vi "Mass_1_3.vi"() -> ()   [LabVIEW 2020]
uses:
  Support/Controls/Cmd_Mouse Popup.ctl
  Support/Controls/Clst_Initialize Input.ctl
  Support/Controls/Clst_Result inspec.ctl
  Support/Controls/Cmd_Var Data IO.ctl
  Variables/Global_Cal Info.vi
panel:
  in  "Measured_ADJ":string[][](table) caption="저울의 지시값 (조정후)"
  out "분동조합":string[][](table)
  in  "Spec 변경":bool
  in  "Random":bool
  out "Spec":string[][](table)
  out "제목":string
  out "편심 오차 시험 분동":string
  out "에러 출력":errorcluster
  out "Condition":string[][](table) caption="2. 직선성 시험"
  in  "최소눈금":string(combo)
  out "단위":string
  out "최대용량":string
  in  "Measured":string[][](table) caption="저울의 지시값"
  in  "Measured 2":string[][](table) caption="1. 편심오차 시험"
  out "Load?":bool
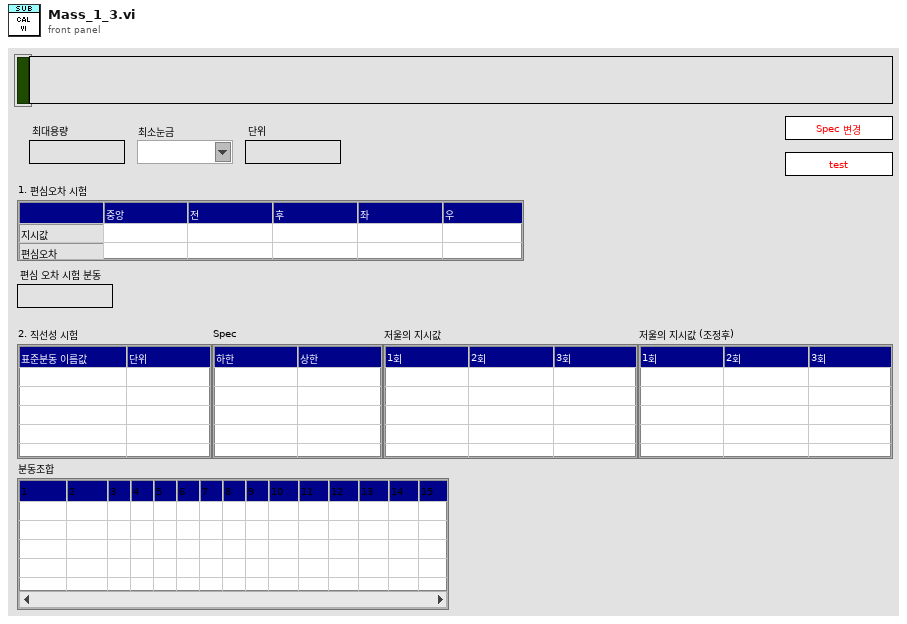
[diagram p1: front panel]
types:
  T1 = typedef "Cmd_Mouse Popup.ctl" = enum16{"활성화", "메뉴선택"}
  T2 = cluster{"Shift":bool, "Ctrl":bool, "Alt":bool, "Cmd":bool, "Opt":bool}
  T3 = typedef "Clst_Initialize Input.ctl" = cluster{"Initialize 1":cluster{"Condition":refnum<vi>[], "Spec":refnum<vi>[], "Measured":refnum<vi>[], "Resolution":refnum<vi>[], "Func_ext":string, "제목":refnum<vi>, "Measured_ADJ":refnum<vi>[]}, "Initialize 2":cluster{"문자열":refnum<vi>[], "콤보박스":refnum<vi>[], "링":refnum<vi>[], "열거형":refnum<vi>[], "테이블":refnum<vi>[], "여러열":refnum<vi>[], "디지털(DBL)":refnum<vi>[], "3D string":refnum<vi>[], "ctrl":refnum<vi>[], "boolean":refnum<vi>[]}}
  T4 = typedef "Clst_Result inspec.ctl" = cluster{"분해능":string, "문자열 1":string, "문자열 2":string, "숫자형 1":i32, "숫자형 2":i32, "숫자형 3":dbl, "문자배열 1D":string[], "문자배열 2D":string[][], "문자배열 3D":string[][][], "문자배열 4D":string[][][][], "불리언 1D":bool[]}
  T5 = typedef "Cmd_Var Data IO.ctl" = enum16{"Condition", "Condition Default", "Condition_Temp", "Resolution", "Resolution Default", "Resolution Old", "Spec", "Spec Default", "Spec Old", "Spec Temp", "Result", "Result2", "Result3", "Result_Temp", "Result_ADJ", "Result_ADJ2", "STD1", "STD2", "STD3", "STD4", "STD5", "STD Temp", "CMC", "CMC Default"}
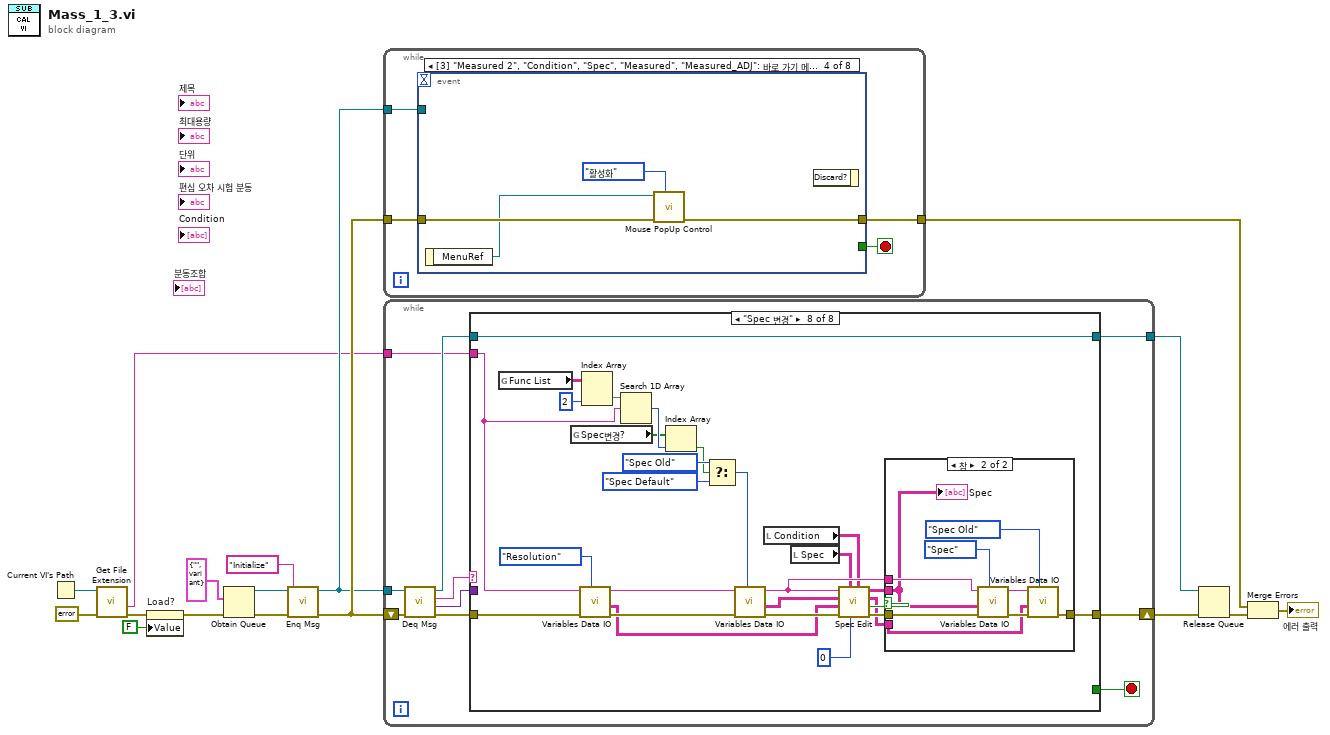
[diagram p0: block diagram]
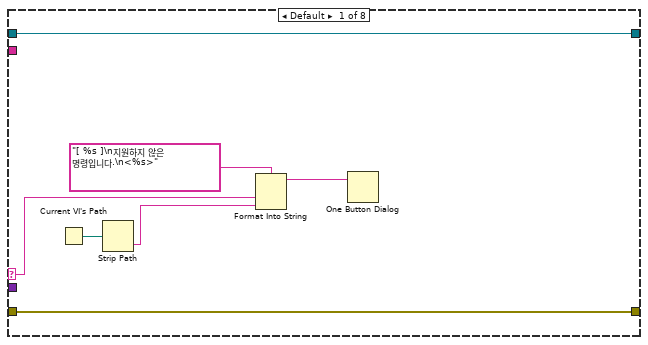
[diagram p2: hidden frame]
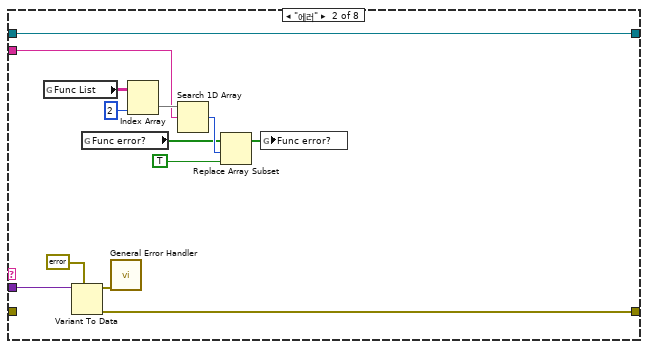
[diagram p3: hidden frame]
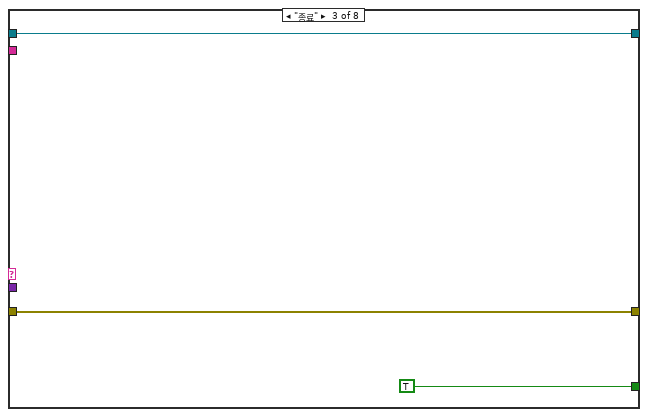
[diagram p4: hidden frame]
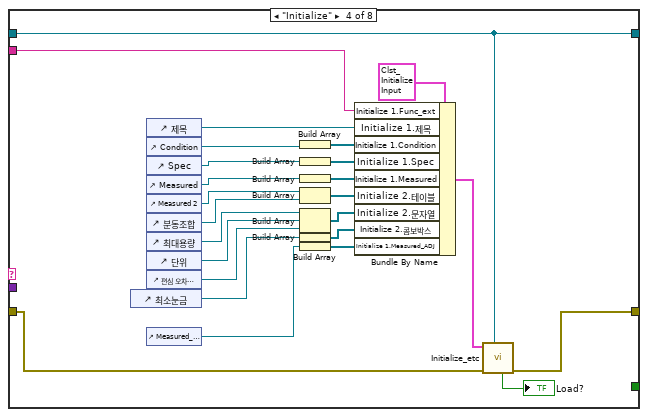
[diagram p5: hidden frame]
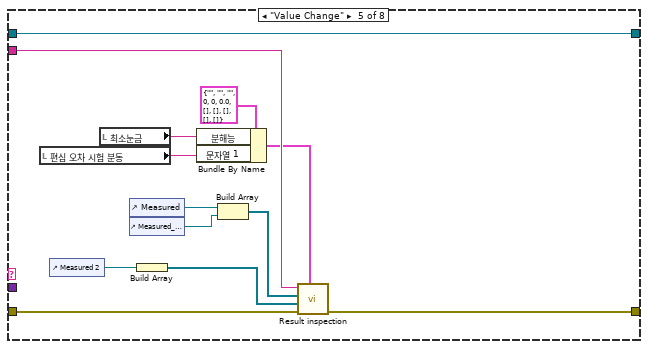
[diagram p6: hidden frame]
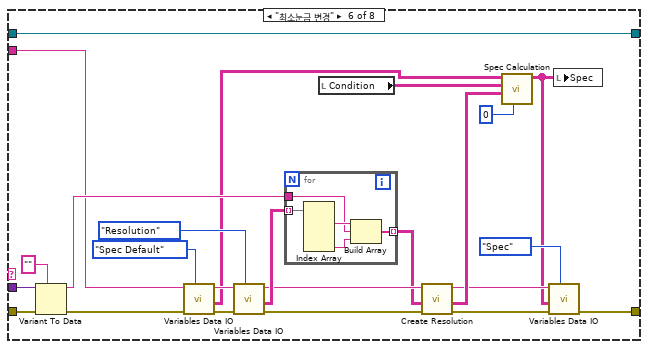
[diagram p7: hidden frame]
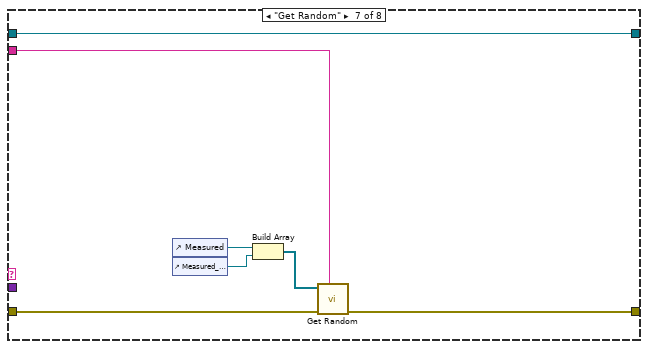
[diagram p8: hidden frame]
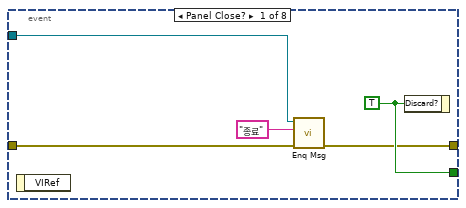
[diagram p10: hidden frame]
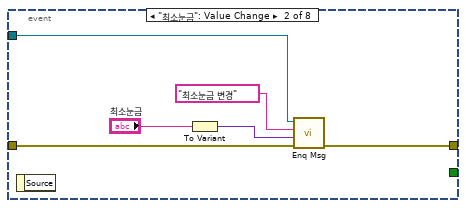
[diagram p11: hidden frame]
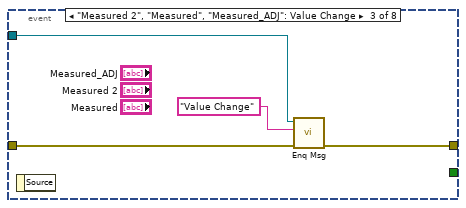
[diagram p12: hidden frame]
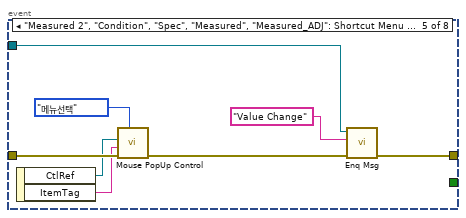
[diagram p13: hidden frame]
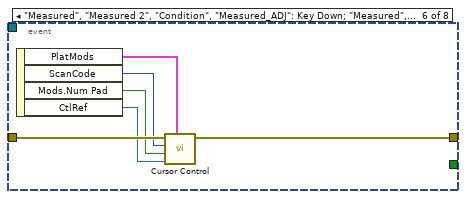
[diagram p14: hidden frame]
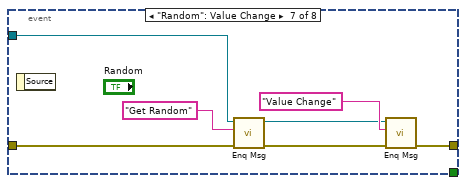
[diagram p15: hidden frame]
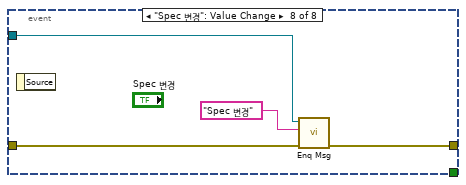
[diagram p16: hidden frame]
diagram:
  n1 = Current VI's Path() -> (path=w5:path)
  n2 = call <vilib>:"Get File Extension.vi"("error in (no error)"=errorcluster {"status"=FALSE, "code"=0, "source"=""} ("에러 상수"), "file"=w5) -> ("error out"=w3:errorcluster, "filename without extension"=w4:string)  [unwired: 5 in, 3 out]
  n3 = property on="Load?" class="Bool (엄격한)"(error in=w3, "Value"=FALSE ("Load?")) -> (error out=w2:errorcluster)  [unwired: 1 in, 1 out]
  n4 = Obtain Queue(element data type=cluster{"메세지":string, "값":variant} {"메세지"="", "값"=variant} ("Message Cluster"), error in (no error)=w2) -> (queue out=w14:refnum<queue>, error out=w16:errorcluster)  [unwired: 3 in, 1 out]
  n5 = call "Enq Msg.vi"("에러 입력(에러 없음)"=w16, "메세지"="Initialize", "큐 입력"=w14) -> ("에러 출력"=w15:errorcluster, "큐 출력"=w12:refnum<queue>)  [unwired: 7 in]
  n6 = while {
    tunnel: w15 -> [w19]
    tunnel: w12 -> [w20]
    tunnel: [w18] -> w9
    stop <- w21 stop-if-true
    n7 = event shown="[3] \"Measured 2\", \"Condition\", \"Spec\", \"Measured\", \"Measured_ADJ\": 바로 가기 메뉴 활성화?" {
      selector: _ -> [_ _ _ _ _ _ _ _]
      dyn-events: _ -> [_ _ _ _ _ _ _ _]
      timeout: _ -> [_ _ _ _ _ _ _ _]
      tunnel: [w26 _ _ _ _ _ _ _] -> w21
      tunnel: w20 -> [w24 w31 w35 _ w42 _ w56 w62]
      tunnel: w19 -> [w25 w32 w36 w39 w47 w54 w57 w64]
      tunnel: [w22 w29 w33 w38 w41 w53 w55 w63] -> w18
      event Panel Close? {
        w26 = TRUE ("버림?")
        n8 = event-data() -> ()  [unwired: 1 in, 1 out]
        n9 = call "Enq Msg.vi"("에러 입력(에러 없음)"=w25, "메세지"="종료", "큐 입력"=w24) -> ("에러 출력"=w22:errorcluster)  [unwired: 7 in, 1 out]
        n10 = event-data("Discard?"=w26) -> ()  [unwired: 1 in, 1 out]
      }
      event "최소눈금": Value Change {
        n11 = event-data() -> ()  [unwired: 1 in, 1 out]
        n12 = To Variant(anything="최소눈금") -> (Variant=w27:variant)
        n13 = call "Enq Msg.vi"("에러 입력(에러 없음)"=w32, "값"=w27, "메세지"="최소눈금 변경", "큐 입력"=w31) -> ("에러 출력"=w29:errorcluster)  [unwired: 6 in, 1 out]
      }
      event "Measured 2", "Measured", "Measured_ADJ": Value Change {
        n14 = event-data() -> ()  [unwired: 1 in, 1 out]
        n15 = call "Enq Msg.vi"("에러 입력(에러 없음)"=w36, "메세지"="Value Change", "큐 입력"=w35) -> ("에러 출력"=w33:errorcluster)  [unwired: 7 in, 1 out]
      }
      event "Measured 2", "Condition", "Spec", "Measured", "Measured_ADJ": Shortcut Menu Activation? {
        n16 = event-data() -> ("MenuRef"=w37:refnum<k9>)  [unwired: 1 in]
        n17 = call "Mouse PopUp Control.vi"("type"=Cmd_Mouse_Popup."활성화", "error in"=w39, "메뉴 참조"=w37) -> ("error out"=w38:errorcluster)  [unwired: 8 in]
        n18 = event-data() -> ()  [unwired: 2 in, 1 out]
      }
      event "Measured 2", "Condition", "Spec", "Measured", "Measured_ADJ": Shortcut Menu Selection (User) {
        n19 = event-data() -> ("CtlRef"=w45:refnum<vi>, "ItemTag"=w46:string)  [unwired: 1 in]
        n20 = call "Mouse PopUp Control.vi"("type"=Cmd_Mouse_Popup."메뉴선택", "error in"=w47, "아이템 태그"=w46, "Tbl 참조 번호"=w45) -> ("error out"=w43:errorcluster)  [unwired: 7 in]
        n21 = call "Enq Msg.vi"("에러 입력(에러 없음)"=w43, "메세지"="Value Change", "큐 입력"=w42) -> ("에러 출력"=w41:errorcluster)  [unwired: 7 in, 1 out]
      }
      event "Measured", "Measured 2", "Condition", "Measured_ADJ": Key Down; "Measured", "Measured 2", "Condition", "Measured_ADJ": Key Repeat {
        n22 = event-data() -> ("PlatMods"=w49:T2, "ScanCode"=w52:i16, "Mods.Num Pad"=w51:bool, "CtlRef"=w50:refnum<vi>)  [unwired: 1 in]
        n23 = call "Cursor Control.vi"("플랫폼 조합키"=w49, "참조"=w50, "Num Pad"=w51, "ScanCode"=w52, "error in"=w54) -> ("error out"=w53:errorcluster)  [unwired: 5 in, 1 out]
      }
      event "Random": Value Change {
        n24 = event-data() -> ()  [unwired: 1 in, 1 out]
        n25 = call "Enq Msg.vi"("에러 입력(에러 없음)"=w57, "메세지"="Get Random", "큐 입력"=w56) -> ("에러 출력"=w59:errorcluster, "큐 출력"=w60:refnum<queue>)  [unwired: 7 in]
        n26 = call "Enq Msg.vi"("에러 입력(에러 없음)"=w59, "메세지"="Value Change", "큐 입력"=w60) -> ("에러 출력"=w55:errorcluster)  [unwired: 7 in, 1 out]
      }
      event "Spec 변경": Value Change {
        n27 = event-data() -> ()  [unwired: 1 in, 1 out]
        n28 = call "Enq Msg.vi"("에러 입력(에러 없음)"=w64, "메세지"="Spec 변경", "큐 입력"=w62) -> ("에러 출력"=w63:errorcluster)  [unwired: 7 in, 1 out]
      }
    }
  }
  n29 = while {
    shift-right: [w75] -> w11
    shift-left: w15 -> [w74]
    tunnel: w12 -> [w72]
    tunnel: [w67] -> w10
    tunnel: w4 -> [w66]
    stop <- w68 stop-if-true
    n30 = call "Deq Msg.vi"("에러 입력(에러 없음)"=w74, "큐 입력"=w72) -> ("에러 출력"=w73:errorcluster, "값"=w69:variant, "메세지"=w71:string, "큐 출력"=w70:refnum<queue>)  [unwired: 6 in]
    n31 = case shown="\"Spec 변경\"" w71 {
      selector: w71 -> [w78 _ _ _ _ _ _ _]
      tunnel: w73 -> [w82 _ w98 w104 w129 w158 w170 w193]
      tunnel: [w82 w92 w98 w103 w135 w139 w169 w197] -> w75
      tunnel: w70 -> [w81 w91 w96 w105 w136 w160 w172 w199]
      tunnel: w69 -> [_ w93 _ _ _ w157 _ _]
      tunnel: [_ _ TRUE ("버림?") _ _ _ _ _] -> w68
      tunnel: [w81 w91 w96 w105 w136 w160 w172 w199] -> w67
      tunnel: w66 -> [_ w83 _ w106 w134 w149 w167 w174]
      frame Default {
        n32 = Current VI's Path() -> (path=w77:path)
        n33 = Strip Path(path=w77) -> (name=w76:string)  [unwired: 1 out]
        n34 = Format Into String(format string="[ %s ]\n지원하지 않은 명령입니다.\n<%s>" ("메시지"), w78, w76) -> (resulting string=w79:string)  [unwired: 2 in, 1 out]
        n35 = One Button Dialog(message=w79) -> ()  [unwired: 1 in, 1 out]
      }
      frame "에러" {
        n36 = global read "Global_Cal Info.vi" "Func List"() -> (w85:string[][])
        n37 = Variant To Data(type=errorcluster {"status"=FALSE, "code"=0, "source"=""} ("에러 출력"), Variant=w93) -> (data=w95:errorcluster, error out=w92:errorcluster)  [unwired: 1 in]
        n38 = global read "Global_Cal Info.vi" "Func error?"() -> (w88:bool[])
        n39 = call <vilib>:"General Error Handler.vi"("error in (no error)"=w95) -> ()  [unwired: 10 in, 5 out]
        n40 = Index Array(array=w85, index (col)=2 ("비활성화된 인덱스 (열)")) -> (element=w86:string[])  [unwired: 1 in]
        n41 = Search 1D Array(1D array=w86, element=w83) -> (index of element=w89:i32)  [unwired: 1 in]
        n42 = Replace Array Subset(array=w88, new element=TRUE ("새 원소/부분배열"), index=w89) -> (w90:bool[])
        n43 = global write "Global_Cal Info.vi" "Func error?"(w90) -> ()
      }
      frame "종료" {
      }
      frame "Initialize" {
        n44 = control-ref of="최소눈금"() -> (w114:refnum<vi>)
        n45 = control-ref of="제목"() -> (w112:refnum<vi>)
        n46 = control-ref of="Condition"() -> (w121:refnum<vi>)
        n47 = control-ref of="Spec"() -> (w108:refnum<vi>)
        n48 = control-ref of="Measured"() -> (w118:refnum<vi>)
        n49 = control-ref of="Measured 2"() -> (w117:refnum<vi>)
        n50 = control-ref of="분동조합"() -> (w102:refnum<vi>)
        n51 = control-ref of="최대용량"() -> (w111:refnum<vi>)
        n52 = control-ref of="단위"() -> (w110:refnum<vi>)
        n53 = control-ref of="편심 오차 시험 분동"() -> (w109:refnum<vi>)
        n54 = control-ref of="Measured_ADJ"() -> (w101:refnum<vi>)
        n55 = Build Array(w121) -> (w120:refnum<vi>[])
        n56 = Build Array(w108) -> (w107:refnum<vi>[])
        n57 = Build Array(w118) -> (w119:refnum<vi>[])
        n58 = Build Array(w117, w102) -> (w116:refnum<vi>[])
        n59 = Build Array(w111, w110, w109) -> (w115:refnum<vi>[])
        n60 = Build Array(w114) -> (w113:refnum<vi>[])
        n61 = Build Array(w101) -> (w100:refnum<vi>[])
        n62 = Bundle By Name(cluster=T3 {"Initialize 1"={"Condition"=[], "Spec"=[], "Measured"=[], "Resolution"=[], "Func_ext"="", "제목"=refnum, "Measured_ADJ"=[]}, "Initialize 2"={"문자열"=[], "콤보박스"=[], "링"=[], "열거형"=[], "테이블"=[], "여러열"=[], "디지털(DBL)"=[], "3D string"=[], "ctrl"=[], "boolean"=[]}} ("입력 클러스터"), "Initialize 1.Func_ext"=w106, "Initialize 1.제목"=w112, "Initialize 1.Condition"=w120, "Initialize 1.Spec"=w107, "Initialize 1.Measured"=w119, "Initialize 2.테이블"=w116, "Initialize 2.문자열"=w115, "Initialize 2.콤보박스"=w113, "Initialize 1.Measured_ADJ"=w100) -> (w122:T3)
        n63 = call "Initialize_etc.vi"("큐 입력"=w105, "error in"=w104, "입력 클러스터"=w122) -> ("error out"=w103:errorcluster, "Load?"=→"Load?":bool)  [unwired: 6 in, 1 out]
      }
      frame "Value Change" {
        n64 = local read "편심 오차 시험 분동"() -> (w125:string)
        n65 = control-ref of="Measured 2"() -> (w130:refnum<vi>)
        n66 = local read "최소눈금"() -> (w127:string)
        n67 = control-ref of="Measured"() -> (w133:refnum<vi>)
        n68 = control-ref of="Measured_ADJ"() -> (w124:refnum<vi>)
        n69 = Build Array(w130) -> (w131:refnum<vi>[])
        n70 = Bundle By Name(cluster=T4 {"분해능"="", "문자열 1"="", "문자열 2"="", "숫자형 1"=0, "숫자형 2"=0, "숫자형 3"=0.0, "문자배열 1D"=[], "문자배열 2D"=[], "문자배열 3D"=[], "문자배열 4D"=[], "불리언 1D"=[]} ("입력 클러스터"), "분해능"=w127, "문자열 1"=w125) -> (w126:T4)
        n71 = Build Array(w133, w124) -> (w132:refnum<vi>[])
        n72 = call "Result inspection.vi"("입력 클러스터"=w126, "error in"=w129, "Ref. Data (excluded)"=w131, "Ref. Data (Inspection)"=w132, "Func ext"=w134) -> ("error out"=w135:errorcluster)  [unwired: 3 in, 3 out]
      }
      frame "최소눈금 변경" {
        n73 = Variant To Data(error in=w158, type="", Variant=w157) -> (data=w155:string, error out=w150:errorcluster)
        n74 = call "Variables Data IO.vi"("Select"=Cmd_Var_Data_IO."Spec Default", "error in"=w150, "Func_ext"=w149) -> ("error out"=w147:errorcluster, "Data Out"=w145:string[][], "Func_ext Out"=w148:string)  [unwired: 6 in]
        n75 = call "Variables Data IO.vi"("Select"=Cmd_Var_Data_IO."Resolution", "error in"=w147, "Func_ext"=w148) -> ("error out"=w153:errorcluster, "Data Out"=w159:string[][], "Func_ext Out"=w152:string)  [unwired: 6 in]
        n76 = for {
          tunnel: w159 -> [w165] mode=indexing
          tunnel: w155 -> [w163]
          tunnel: [w161] -> w137 mode=indexing
          n77 = Index Array(array=w165) -> (element #1=w164:string, element #4=w162:string)  [unwired: 4 in, 2 out]
          n78 = Build Array(w164, w163, w162) -> (w161:string[])
        }
        n79 = local read "Condition"() -> (w144:string[][])
        n80 = call "Create Resolution.vi"("에러 입력(에러 없음)"=w153, "Resolution"=w137, "Func_ext"=w152) -> ("에러 출력"=w140:errorcluster, "Resolution Out"=w151:string[][], "Func_ext 출력"=w141:string)  [unwired: 6 in]
        n81 = call "Spec Calculation.vi"("기준값 열번호"=0 ("열번호(기준값)"), "Resolution"=w151, "Condition in"=w144, "Spec Default"=w145) -> ("Spec out"=w138:string[][])  [unwired: 6 in, 1 out]
        n82 = call "Variables Data IO.vi"("Select"=Cmd_Var_Data_IO."Spec", "error in"=w140, "Data In"=w138, "Func_ext"=w141) -> ("error out"=w139:errorcluster)  [unwired: 5 in, 2 out]
        n83 = local write "Spec"(w138) -> ()
      }
      frame "Get Random" {
        n84 = control-ref of="Measured"() -> (w168:refnum<vi>)
        n85 = control-ref of="Measured_ADJ"() -> (w166:refnum<vi>)
        n86 = Build Array(w168, w166) -> (w171:refnum<vi>[])
        n87 = call "Get Random.vi"("Func_Ext"=w167, "에러 입력"=w170, "Meas"=w171) -> ("에러 출력"=w169:errorcluster)  [unwired: 7 in, 1 out]
      }
      frame "Spec 변경" {
        n88 = global read "Global_Cal Info.vi" "Func List"() -> (w179:string[][])
        n89 = global read "Global_Cal Info.vi" "Spec변경?"() -> (w175:bool[])
        n90 = call "Variables Data IO.vi"("Select"=Cmd_Var_Data_IO."Resolution", "error in"=w193, "Func_ext"=w174) -> ("error out"=w192:errorcluster, "Data Out"=w186:string[][], "Func_ext Out"=w191:string)  [unwired: 6 in]
        n91 = Index Array(array=w179, index (col)=2 ("비활성화된 인덱스 (열)")) -> (element=w177:string[])  [unwired: 1 in]
        n92 = Search 1D Array(1D array=w177, element=w174) -> (index of element=w176:i32)  [unwired: 1 in]
        n93 = Index Array(array=w175, index=w176) -> (element=w180:bool)
        n94 = Select(t=Cmd_Var_Data_IO."Spec Old" ("Select"), s=w180, f=Cmd_Var_Data_IO."Spec Default" ("Select")) -> (s? t:f=w173:T5)
        n95 = call "Variables Data IO.vi"("Select"=w173, "error in"=w192, "Func_ext"=w191) -> ("error out"=w194:errorcluster, "Data Out"=w185:string[][], "Func_ext Out"=w187:string)  [unwired: 6 in]
        n96 = local read "Condition"() -> (w183:string[][])
        n97 = local read "Spec"() -> (w184:string[][])
        n98 = call "Spec Edit.vi"("Condition"=w183, "열번호(기준값)"=0 ("기준열(0)"), "Spec Value"=w184, "에러 입력(에러 없음)"=w194, "Resolution"=w186, "Spec Default"=w185, "Func_ext"=w187) -> ("에러 출력"=w198:errorcluster, "변경?"=w195:bool, "Spec Default out"=w189:string[][], "Spec 출력"=w196:string[][])  [unwired: 1 in]
        n99 = case shown="참" w195 {
          tunnel: w198 -> [w200 w208]
          tunnel: [w200 w204] -> w197
          tunnel: w196 -> [_ w206]
          tunnel: w187 -> [_ w207]
          tunnel: w189 -> [_ w202]
          frame False {
          }
          frame True {
            n100 = call "Variables Data IO.vi"("Select"=Cmd_Var_Data_IO."Spec", "error in"=w208, "Data In"=w206, "Func_ext"=w207) -> ("error out"=w205:errorcluster, "Func_ext Out"=w203:string)  [unwired: 5 in, 1 out]
            n101 = call "Variables Data IO.vi"("Select"=Cmd_Var_Data_IO."Spec Old", "error in"=w205, "Data In"=w202, "Func_ext"=w203) -> ("error out"=w204:errorcluster)  [unwired: 5 in, 2 out]
            "Spec" <- w206
          }
        }
      }
    }
  }
  n102 = Release Queue(queue=w10, error in (no error)=w11) -> (error out=w8:errorcluster)  [unwired: 1 in, 2 out]
  n103 = Merge Errors(w9, w8) -> (→"에러 출력":errorcluster)
